vi "Destroy Self.vi"(7 "Sender":refnum<class "Sender.lvclass">, 11 "Destroy Self in":refnum<class "Destroy Self.lvclass">) -> (0 "Error out":errorcluster, 3 "Destroy Self out":refnum<class "Destroy Self.lvclass">)   [LabVIEW 2025, in "jettl.lvlib" / "Destroy Self Msg.lvlib" / "Destroy Self.lvclass"]
uses:
  Destroy Self.lvclass
  Sender/Sender/Sender.lvclass
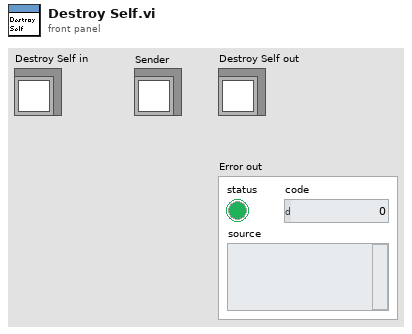
[diagram p1: front panel]
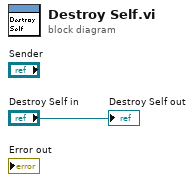
[diagram p0: block diagram]
diagram:
  "Destroy Self out" <- "Destroy Self in"
